vi "Lake Shore 335 Acquire Multiple Readings.vi"(0 "VISA resource name":refnum<visa-resource-name>) -> ()   [LabVIEW 2015]
doc: "This example VI demonstrates the proper use of the Sensor Data (Multiple Readings) VI. This VI reads and returns multiple sensor readings from the instrument. Control over interval between readings is also provided."
uses:
  Public/Data/Sensor Data (Multiple Readings).vi
  Lake Shore 335.lvlib
panel:
  in  "Input (0:A)":u16(ring) items=["A", "B"]
  in  "Data Source (0:Kelvin)":u16(ring) items=["Kelvin", "Celsius", "Sensor Units"]
  in  "Reading Interval (100)":dbl=100.0
  in  "Sample Count (1)":i32=1
  out "Sensor Data":dbl[](array[numeric]) format="%.4f"
  in  "Serial Configuration":T1={"Baud Rate"=57600, "Parity"=1, "Data Bits"=7, "Stop Bits"=10, "Flow Control"=0} {"Flow Control" items=["None", "XON/XOFF", "RTS/CTS", "XON/XOFF & RTS/CTS", "DTR/DSR", "XON/XOFF & DTR/DSR"]; "Stop Bits" items=["1.0"=10, "1.5"=15, "2.0"=20]; "Data Bits" items=["7"=7, "8"=8]; "Parity" items=["None", "Odd", "Even", "Mark", "Space"]; "Baud Rate" items=["300"=300, "600"=600, "1200"=1200, "2400"=2400, "4800"=4800, "9600"=9600, "19200"=19200, "38400"=38400, "57600"=57600]}
  # "(c) 2011 Lake Shore Cryotronics Inc.  ALL RIGHTS RESERVED."
  # "Sensor Data"
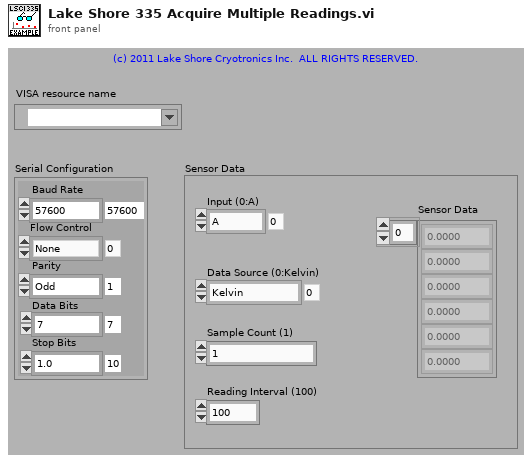
[diagram p1: front panel]
types:
  T1 = cluster{"Baud Rate":u32, "Parity":u16, "Data Bits":u16, "Stop Bits":u16, "Flow Control":u16}
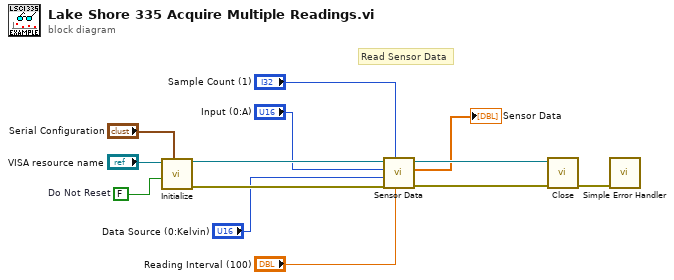
[diagram p0: block diagram]
diagram:
  w11 = FALSE  # Do Not Reset
  # "Read Sensor Data"
  n1 = call "Initialize.vi"("Serial Configuration"="Serial Configuration", "Reset (True)"=w11, "VISA resource name"="VISA resource name") -> ("error out"=w6:errorcluster, "VISA resource name out"=w7:refnum<visa-resource-name>)  [unwired: 7 in]
  n2 = call-poly "Sensor Data.vi"("Reading Interval (100)"="Reading Interval (100)", "Sample Count (1)"="Sample Count (1)", "error in (no error)"=w6, "Data Source (0:Kelvin)"="Data Source (0:Kelvin)", "Input (0:A)"="Input (0:A)", "VISA resource name"=w7) -> ("error out"=w8:errorcluster, "Sensor Data"=→"Sensor Data":dbl[], "VISA resource name out"=w9:refnum<visa-resource-name>)  [unwired: 3 in]
  n3 = call "Close.vi"("error in (no error)"=w8, "VISA resource name"=w9) -> ("error out"=w12:errorcluster)  [unwired: 9 in]
  n4 = call <vilib>:"Simple Error Handler.vi"("error in (no error)"=w12) -> ()  [unwired: 4 in, 5 out]
